vi "Host Window.vi"(8 "error in (no error)":errorcluster, 10 "Child Hwnd":u32, 11 "Parent Hwnd":i32) -> (0 "error out":errorcluster)   [LabVIEW 2016, in "LV MDI.lvclass"]
doc: "Set Parent Window to the specified window."
uses:
  LV MDI.lvclass
  user32.dll
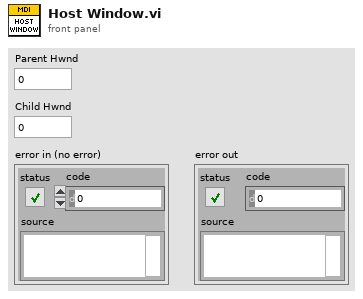
[diagram p1: front panel]
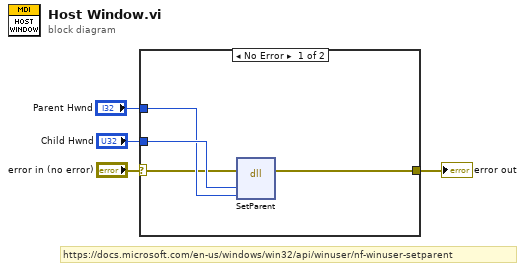
[diagram p0: block diagram]
diagram:
  # "https://docs.microsoft.com/en-us/windows/win32/api/winuser/nf-winuser-setparent"
  n1 = case shown="No Error" "error in (no error)" {
    selector: "error in (no error)" -> [w5 w9]
    tunnel: [w8 w9] -> w4
    tunnel: "Child Hwnd" -> [w7 _]
    tunnel: "Parent Hwnd" -> [w6 _]
    frame No Error {
      n2 = dll-call lib="user32.dll" fn="SetParent"(error in=w5, "Child"=w7, "NewParent"=w6) -> (error out=w8:errorcluster)  [unwired: 5 in, 1 out]
    }
    frame Error {
    }
  }
  "error out" <- w4
